vi "lqManifestation.vi"(11 "LQSerialData in":refnum<class "LQSerialData.lvclass">) -> (2 "Manifestation":string, 3 "LQSerialData out":refnum<class "LQSerialData.lvclass">)   [LabVIEW 2014, in "LQ Core.lvlib" / "LQSerialData.lvclass"]
uses:
  LQSerialData.lvclass
  LQSerialData.lvclass/LQSerialData.ctl
panel:
  # "Copyright (c) 2016 Sze Howe Koh\n\nThis Source Code Form is subject to the terms of the Mozilla Public\nLicense, v. 2.0. If a copy of the MPL was not distributed with this\nfile, You can obtain one at http://mozilla.org/MPL/2.0/."
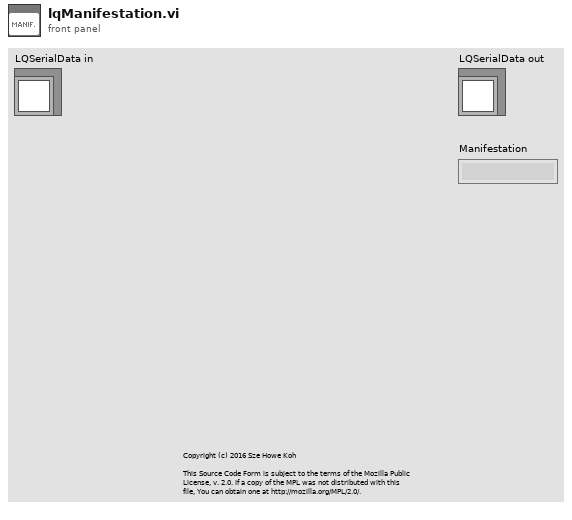
[diagram p1: front panel]
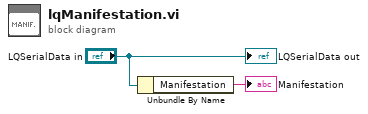
[diagram p0: block diagram]
diagram:
  n1 = Unbundle By Name("LQSerialData in") -> ("Manifestation"=→"Manifestation":string)
  "LQSerialData out" <- "LQSerialData in"
